vi "Test.vi"(8 "stop":bool, 11 "timeout [ms]":i32=33) -> (0 "error out":errorcluster, 2 "message":string, 3 "time [ms]":u32)   [LabVIEW 2022 SP3, in "Logger.lvlib"]
uses:
  Logger.lvlib
  Logger/_Level.ctl
  FileHandler/FileHandler.lvclass
  C:/Users/jakub/repos/gh/sw4sys/lv-logger/Logger/Source/Handler/Handler.lvclass
  Logger/Logger.lvclass
  DateTime/Source/DateTime.lvlib
  Handler/Handler.lvclass
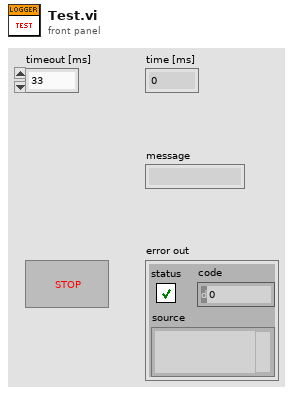
[diagram p1: front panel]
types:
  T1 = typedef "Logger.lvlib/Logger.lvclass/_Level.ctl" = enum16{"NOTSET", "DEBUG", "INFO", "WARNING", "ERROR", "CRITICAL"}
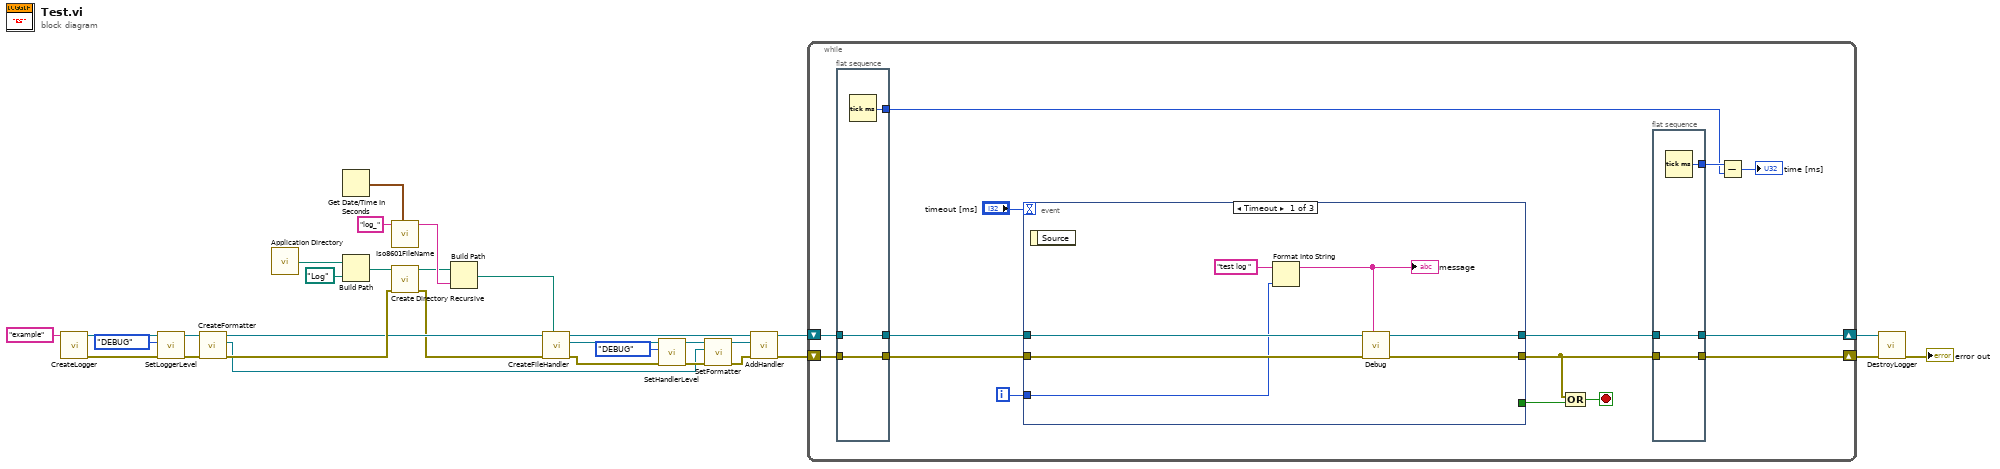
[diagram p0: block diagram]
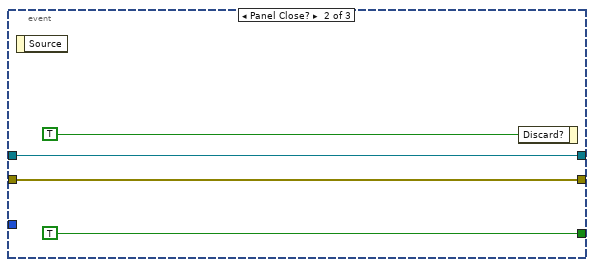
[diagram p2: hidden frame]
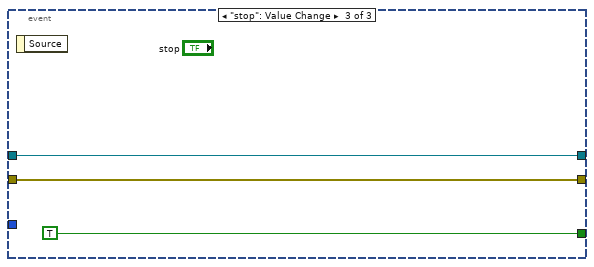
[diagram p3: hidden frame]
diagram:
  n1 = call "CreateLogger.vi"("Name"="example") -> ("error out"=w31:errorcluster, "Logger"=w23:refnum<class "Logger.lvclass">)  [unwired: 9 in]
  n2 = call-dynamic "SetLoggerLevel.vi"("error in (no error)"=w31, "Level"=_Level."DEBUG", "Logger in"=w23) -> ("error out"=w24:errorcluster, "Logger out"=w19:refnum<class "Logger.lvclass">)  [unwired: 7 in]
  n3 = call-dynamic "CreateFormatter.vi"("error in (no error)"=w24, "Logger in"=w19) -> ("error out"=w16:errorcluster, "Formatter"=w3:refnum<class "Formatter.lvclass">, "Logger out"=w11:refnum<class "Logger.lvclass">)  [unwired: 7 in]
  n4 = call <vilib>:"Application Directory.vi"() -> ("Application Directory"=w28:path)
  n5 = Get Date/Time In Seconds() -> (seconds since 1Jan1904=w5:timestamp)
  n6 = Build Path(base path=w28, name or relative path=path "Log") -> (appended path=w14:path)
  n7 = call "Iso8601FileName.vi"("TimeStamp"=w5, "Prefix ('')"="log_") -> ("FileName"=w13:string)  [unwired: 9 in]
  n8 = call <vilib>:"Create Directory Recursive.vi"("error in (no error)"=w16, "directory"=w14) -> ("error out"=w10:errorcluster, "directory copy"=w4:path)  [unwired: 3 in, 1 out]
  n9 = Build Path(base path=w4, name or relative path=w13) -> (appended path=w12:path)
  n10 = call-dynamic "CreateFileHandler.vi"("FIlePath"=w12, "error in (no error)"=w10, "Logger in"=w11) -> ("error out"=w29:errorcluster, "FileHandler"=w9:refnum<class "FileHandler.lvclass">, "Logger out"=w7:refnum<class "Logger.lvclass">)  [unwired: 6 in]
  n11 = call "SetHandlerLevel.vi"("error in (no error)"=w29, "Level"=_Level."DEBUG", "Handler in"=w9) -> ("error out"=w25:errorcluster, "Handler out"=w8:refnum<class "Handler.lvclass">)  [unwired: 7 in]
  n12 = call "SetFormatter.vi"("error in (no error)"=w25, "Formatter in"=w3, "Handler in"=w8) -> ("error out"=w18:errorcluster, "Handler out"=w17:refnum<class "Handler.lvclass">)  [unwired: 6 in, 1 out]
  n13 = call-dynamic "AddHandler.vi"("error in (no error)"=w18, "Handler in"=w17, "Logger in"=w7) -> ("error out"=w21:errorcluster, "Logger out"=w20:refnum<class "Logger.lvclass">)  [unwired: 6 in, 1 out]
  n14 = while {
    shift-right: [w35] -> w26
    shift-left: w20 -> [w39]
    shift-right: [w37] -> w27
    shift-left: w21 -> [w41]
    i -> [w43]
    stop <- w45 stop-if-true
    n15 = flat-sequence {
      tunnel: [w52] -> w42
      tunnel: w41 -> [w52]
      tunnel: [w51] -> w40
      tunnel: w39 -> [w51]
      tunnel: [w50] -> w33
      frame #0 {
        n16 = Tick Count (ms)() -> (millisecond timer value=w50:u32)
      }
    }
    n17 = event shown="[0] Timeout" {
      selector: _ -> [_ _ _]
      dyn-events: _ -> [_ _ _]
      timeout: "timeout [ms]" -> [_ _ _]
      tunnel: w40 -> [w59 w62 w66]
      tunnel: w42 -> [w58 w61 w65]
      tunnel: [w57 w62 w66] -> w36
      tunnel: [_ TRUE ("stop") TRUE ("stop")] -> w46
      tunnel: [w55 w61 w65] -> w38
      tunnel: w43 -> [w53 _ _]
      event Timeout {
        n18 = event-data() -> ()  [unwired: 1 in, 1 out]
        n19 = Format Into String(initial string="test log ", w53) -> (resulting string=w54:string)  [unwired: 2 in, 1 out]
        "message" <- w54
        n20 = call-dynamic "Debug.vi"("Message"=w54, "error in (no error)"=w58, "Logger in"=w59) -> ("error out"=w55:errorcluster, "Logger out"=w57:refnum<class "Logger.lvclass">)  [unwired: 7 in]
      }
      event Panel Close? {
        n21 = event-data() -> ()  [unwired: 1 in, 1 out]
        n22 = event-data("Discard?"=TRUE) -> ()  [unwired: 1 in, 1 out]
      }
      event "stop": Value Change {
        n23 = event-data() -> ()  [unwired: 1 in, 1 out]
      }
    }
    n24 = Compound Arithmetic op=OR(w38, w46) -> (w45:bool)
    n25 = flat-sequence {
      tunnel: [w49] -> w37
      tunnel: w38 -> [w49]
      tunnel: [w48] -> w35
      tunnel: w36 -> [w48]
      tunnel: [w47] -> w34
      frame #0 {
        n26 = Tick Count (ms)() -> (millisecond timer value=w47:u32)
      }
    }
    n27 = Subtract(x=w34, y=w33) -> (x-y=→"time [ms]":u32)
  }
  n28 = call-dynamic "DestroyLogger.vi"("error in (no error)"=w27, "Logger in"=w26) -> ("error out"=→"error out":errorcluster)  [unwired: 9 in]
